vi "Get Process Variable List.vi"(8 "Error In":errorcluster, 9 "Selected Libraries":i32[](listbox), 10 "library URL":string[](array[string]), 11 "library Name":string[](array[string])) -> (0 "Error Out":errorcluster, 1 "Selected Library Names":string[](array[string]), 2 "Selected Library URLs":string[](array[string]), 3 "Container Variables":T1)   [LabVIEW 2014]
doc: "<B>Copyright</B>: (c) MHWirth 2015. All rights reserved.\n\nThis subVI provides a list of variable information (name + URLs) for the selected deployed process/processes (library/libraries)."
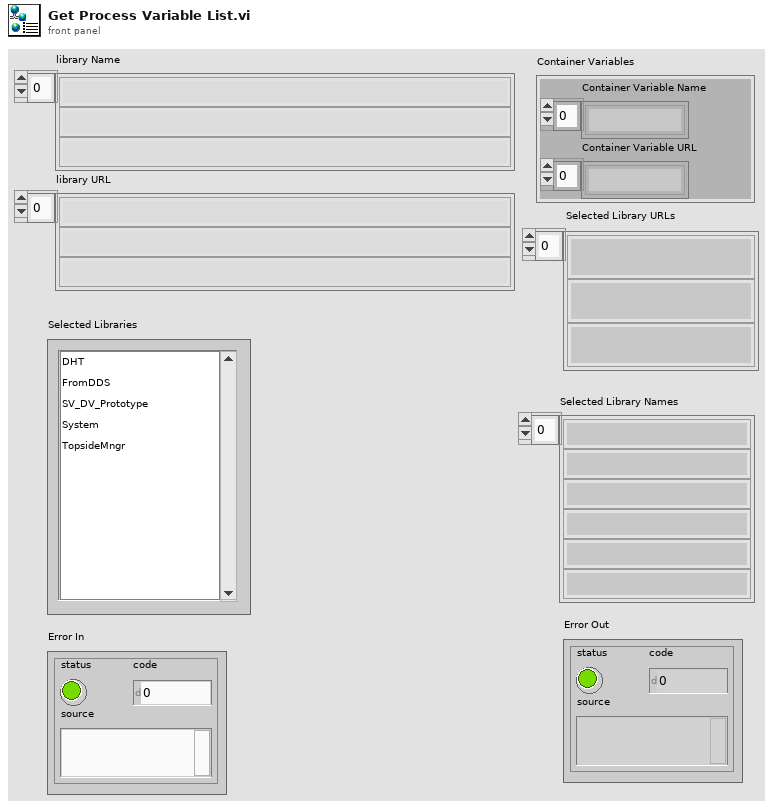
[diagram p1: front panel]
types:
  T1 = cluster{"Container Variable Name":string[], "Container Variable URL":string[]}
  T2 = cluster{"Number of Variables":i32, "Variable/Parent Name array":string[][], "URL array":string[], "Type array":string[]}
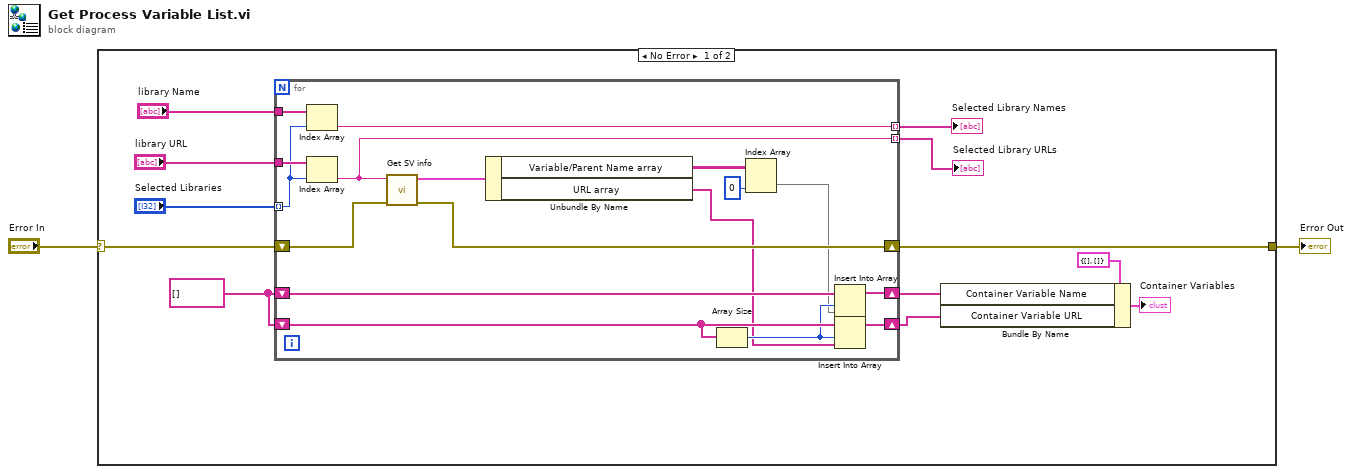
[diagram p0: block diagram]
diagram:
  n1 = case shown="No Error" "Error In" {
    selector: "Error In" -> [w12 w32]
    tunnel: [w6 w32] -> w1
    frame No Error {
      w11 = string[] []
      n2 = for {
        tunnel: "Selected Libraries" -> [w24] mode=indexing
        tunnel: "library URL" -> [w31]
        shift-right: [w19] -> w6
        shift-left: w12 -> [w21]
        shift-right: [w29] -> w9
        shift-left: w11 -> [w30]
        shift-right: [w28] -> w8
        shift-left: w11 -> [w27]
        tunnel: "library Name" -> [w25]
        tunnel: [w23] -> w4 mode=indexing
        tunnel: [w22] -> w3 mode=indexing
        n3 = Index Array(array=w25, index=w24) -> (element=w23:string)
        n4 = Index Array(array=w31, index=w24) -> (element=w22:string)
        n5 = call "Get SV info.vi"("Error In"=w21, "container refnum in"=w22) -> ("Error Out"=w19:errorcluster, "Deployed Shared Variable Information"=w20:T2)  [unwired: 7 in, 1 out]
        n6 = Unbundle By Name(w20) -> ("Variable/Parent Name array"=w17:string[][], "URL array"=w16:string[])
        n7 = Array Size(array=w27) -> (size(s)=w26:i32)
        n8 = Index Array(array=w17, index (col)=0 ("disabled index (col)")) -> (element=w15:string[])  [unwired: 1 in]
        n9 = Insert Into Array(array=w30, index=w26, new element=w15) -> (w29:string[])
        n10 = Insert Into Array(array=w27, index=w26, new element=w16) -> (w28:string[])
      }
      "Selected Library Names" <- w4
      "Selected Library URLs" <- w3
      n11 = Bundle By Name(cluster=T1 {"Container Variable Name"=[], "Container Variable URL"=[]} ("output cluster"), "Container Variable Name"=w9, "Container Variable URL"=w8) -> (→"Container Variables":T1)
    }
    frame Error {
    }
  }
  "Error Out" <- w1
